vi "FIR Filter (CDB).vi"(2 "init/cont (init:F)":bool, 3 "FIR Coefficients":dbl[](array[numeric]), 5 "X":cdb[](array[numeric])) -> (0 "error":i32, 1 "Filtered X":cdb[](array[numeric]))   [LabVIEW 2010, in "NI_AALBase.lvlib"]
doc: "Filters the input sequence<B> X</B> using the direct-form FIR filter specified by <B>FIR Coefficients</B>. Wire data to the <B>X</B> input to determine the polymorphic instance to use or manually select the instance."
uses:
  NI_AALBase.lvlib
  lvanlys.dll
panel:
  # "FIR Filter"
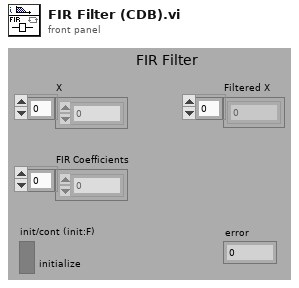
[diagram p1: front panel]
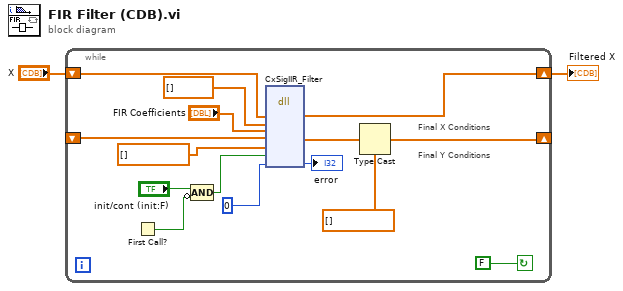
[diagram p0: block diagram]
diagram:
  n1 = while {
    shift-left: _ -> [w12]
    shift-right: [w17] -> _
    shift-right: [w5] -> w1
    shift-left: "X" -> [w6]
    stop <- FALSE continue-if-true
    # "Final Y Conditions"
    # "Final X Conditions"
    n2 = First Call?() -> (First Call?: T/F=w9:bool)
    n3 = Compound Arithmetic op=AND("init/cont (init:F)", invert w9) -> (w7:bool)
    n4 = dll-call lib="C:/Program Files/National Instruments/LabVIEW 2010/resource/lvanlys.*" fn="CxSigIIR_Filter"("X"=w6, "Reverse Coefficients"=dbl[] [], "FIR Coefficients"="FIR Coefficients", "type for the shift register"=w12, "type for the shift register"=cdb[] [], "output param"=w7, "dsperr"=0) -> ("X"=w5:cdb[], "type for the shift register"=w11:cdb[], "dsperr"=→"error":i32)  [unwired: 8 in, 2 out]
    n5 = Type Cast(type=cdb[] [] ("type for the shift register"), x=w11) -> (*(type *) &x=w17:cdb[])
  }
  "Filtered X" <- w1
